vi "Update Script.vi"   [LabVIEW 2018]
doc: "Updates the script periodically. Put this in the disable vi."
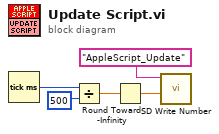
[diagram p0: block diagram]
diagram:
  n1 = Tick Count (ms)() -> (millisecond timer value=w5:u32)
  n2 = Divide(x=w5, y=u32 500) -> (x/y=w3:dbl)
  n3 = Round Toward -Infinity(1:w3) -> (0:w2:dbl)
  n4 = call <vilib>:"SD Write Number.vi"("Numeric"=w2, "Name"="AppleScript_Update") -> ()  [unwired: 8 in, 2 out]
